vi "Host - Thruster Decode (SubVI).vi"(10 "Array":dbl[](array[numeric])=[0.0, 0.0, 0.0, 0.0, 0.0, 0.0, 0.0, 0.0, 0.0, 0.0, 0.0], 11 "read buffer":string) -> (3 "Data init out":dbl[](array[numeric]))   [LabVIEW 2021]
panel:
  out "thruster data":dbl[](array[numeric])
  out "speed":dbl
  out "command 55":u8[](array[numeric])
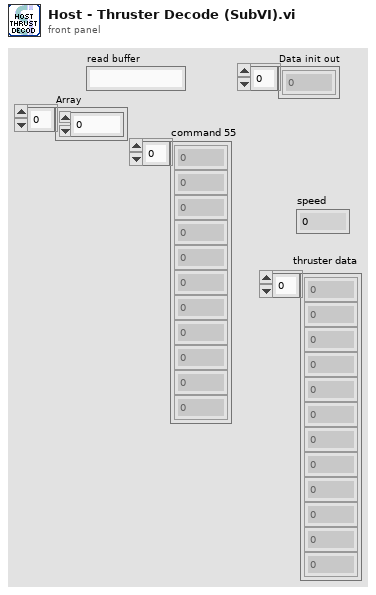
[diagram p1: front panel]
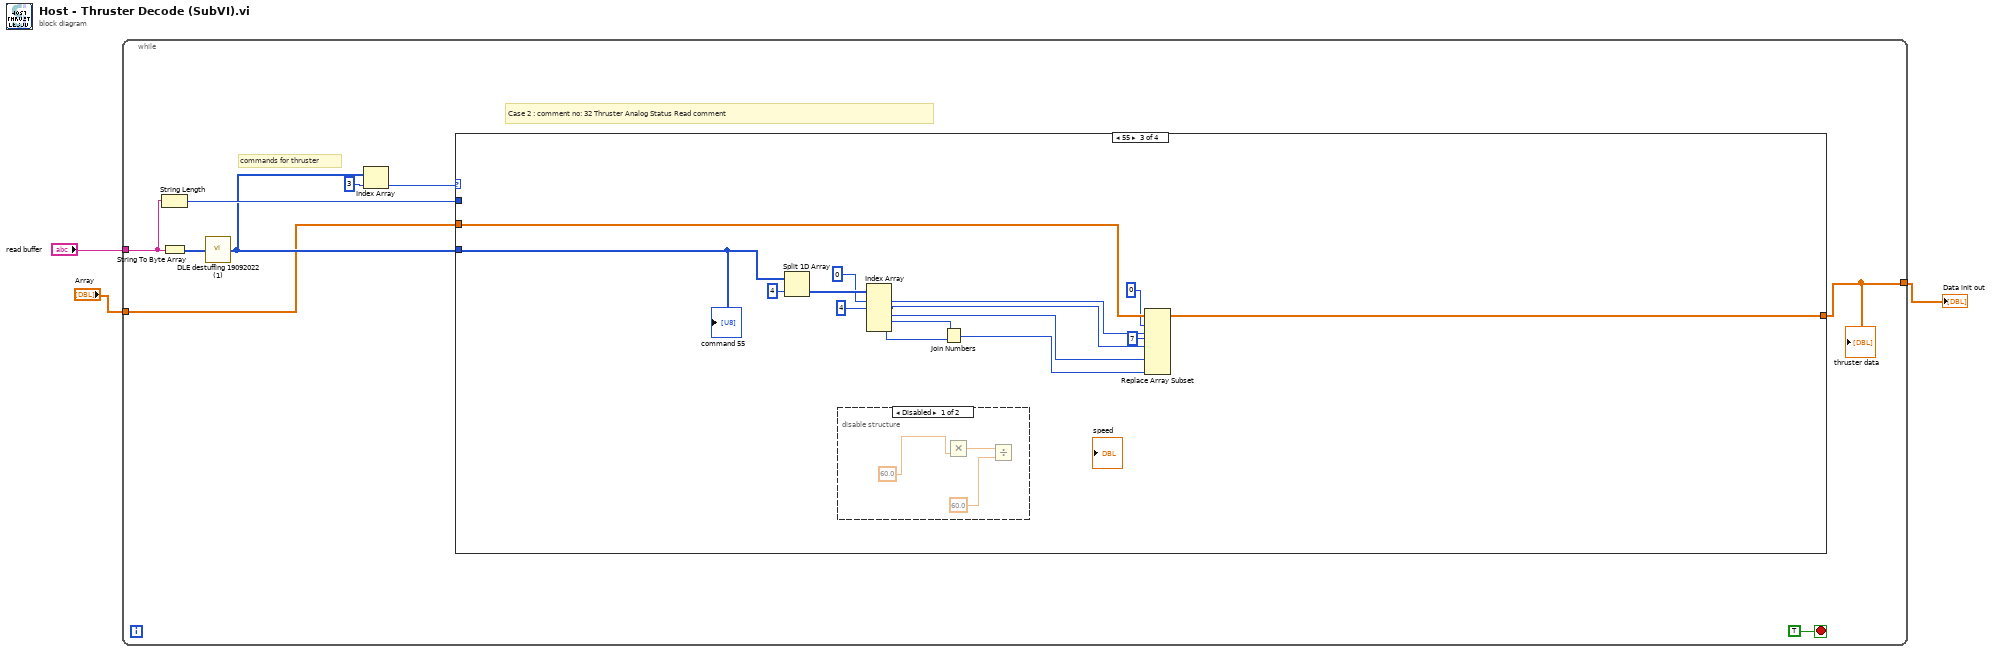
[diagram p0: block diagram]
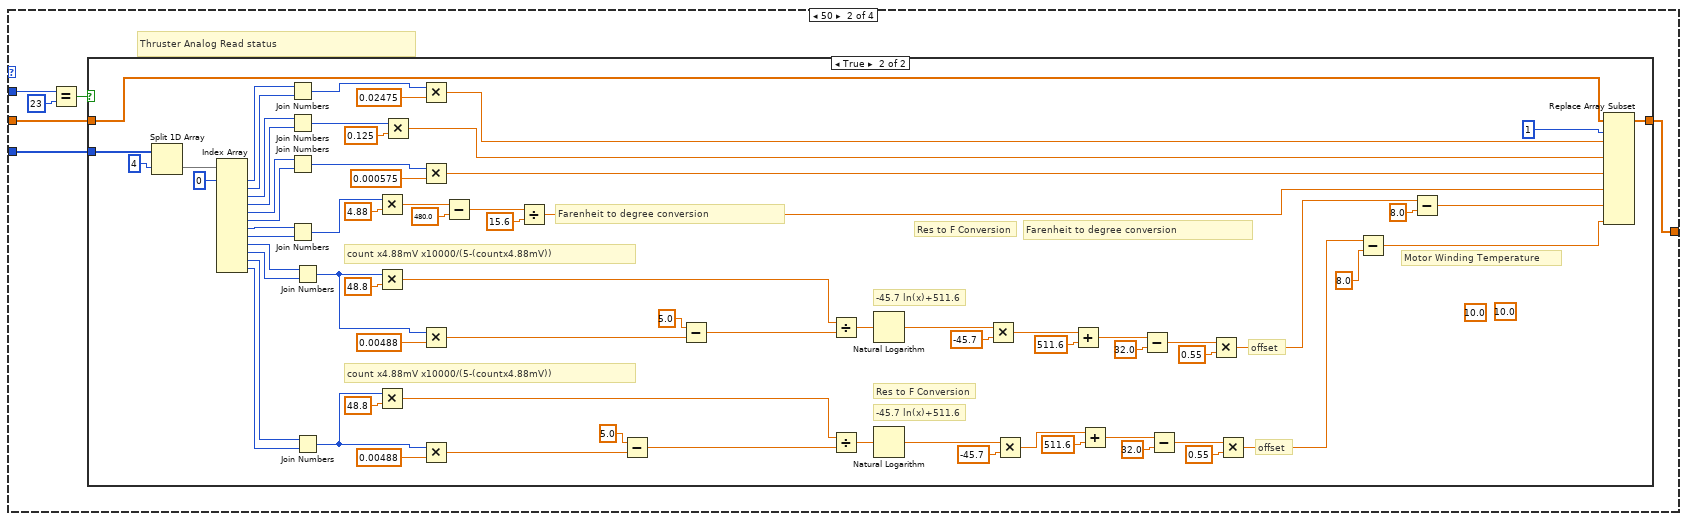
[diagram p3: hidden frame]
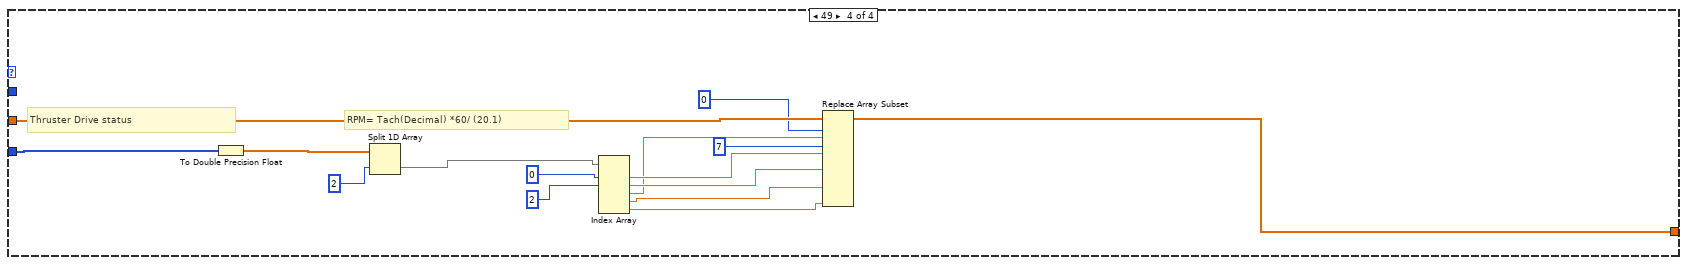
[diagram p6: hidden frame]
diagram:
  n1 = while {
    tunnel: "read buffer" -> [w4]
    tunnel: [w6] -> w2
    tunnel: "Array" -> [w5]
    stop <- TRUE stop-if-true
    # "commands for thruster"
    # "Case 2 : comment no: 32 Thruster Analog Status Read comment"
    n2 = String Length(string=w4) -> (length=w12:i32)
    n3 = String To Byte Array(string=w4) -> (unsigned byte array=w10:u8[])
    n4 = call "DLE destuffing 19092022 (1).vi"("DLE stuffed input"=w10) -> ("DLE destuffed output"=w11:u8[])  [unwired: 4 in]
    n5 = Index Array(array=w11, index=3) -> (element=w8:u8)
    n6 = case shown="55" w8 {
      tunnel: w11 -> [_ w19 w108 w113]
      tunnel: [w13 w17 w96 w125] -> w6
      tunnel: w5 -> [w13 w18 w101 w126]
      tunnel: w12 -> [_ w16 _ _]
      frame 0, Default {
      }
      frame 50 {
        # "Thruster Analog Read status"
        n7 = Equal?(x=w16, y=u32 23) -> (x = y?=w14:bool)
        n8 = case shown="True" w14 {
          tunnel: w19 -> [_ w93]
          tunnel: w18 -> [w20 w30]
          tunnel: [w20 w25] -> w17
          frame False {
          }
          frame True {
            (unwired) 10.0 ("y")
            (unwired) 10.0 ("y")
            # "offset"
            # "-45.7 ln(x)+511.6"
            # "Motor Winding Temperature"
            # "offset"
            # "-45.7 ln(x)+511.6"
            # "Farenheit to degree conversion"
            # "Res to F Conversion"
            # "count x4.88mV x10000/(5-(countx4.88mV))"
            # "Farenheit to degree conversion"
            # "Res to F Conversion"
            # "count x4.88mV x10000/(5-(countx4.88mV))"
            n9 = Split 1D Array(array=w93, index=4) -> (second subarray=w24:u8[])  [unwired: 1 out]
            n10 = Index Array(array=w24, index #1=0 ("index")) -> (element #1=w90:u8, element #2=w89:u8, element #3=w88:u8, element #4=w87:u8, element #5=w86:u8, element #6=w85:u8, element #7=w84:u8, element #8=w83:u8, element #9=w82:u8, element #10=w81:u8, element #11=w80:u8, element #12=w79:u8)  [unwired: 11 in]
            n11 = Join Numbers(hi=w90, lo=w89) -> ((hi.lo)=w78:u16)
            n12 = Join Numbers(hi=w88, lo=w87) -> ((hi.lo)=w76:u16)
            n13 = Join Numbers(hi=w86, lo=w85) -> ((hi.lo)=w74:u16)
            n14 = Join Numbers(hi=w84, lo=w83) -> ((hi.lo)=w72:u16)
            n15 = Join Numbers(hi=w82, lo=w81) -> ((hi.lo)=w32:u16)
            n16 = Join Numbers(hi=w80, lo=w79) -> ((hi.lo)=w31:u16)
            n17 = Multiply(x=w72, y=4.88) -> (x*y=w70:dbl)
            n18 = Multiply(x=w32, y=48.8) -> (x*y=w52:dbl)
            n19 = Multiply(x=w31, y=48.8) -> (x*y=w35:dbl)
            n20 = Multiply(x=w76, y=0.125) -> (x*y=w23:dbl)
            n21 = Multiply(x=w78, y=0.02475) -> (x*y=w22:dbl)
            n22 = Multiply(x=w74, y=0.000575) -> (x*y=w28:dbl)
            n23 = Multiply(x=w32, y=0.00488) -> (x*y=w63:dbl)
            n24 = Multiply(x=w31, y=0.00488) -> (x*y=w46:dbl)
            n25 = Subtract(x=w70, y=480.0) -> (x-y=w68:dbl)
            n26 = Divide(x=w68, y=15.6) -> (x/y=w21:dbl)
            n27 = Subtract(x=5.0, y=w46) -> (x-y=w47:dbl)
            n28 = Subtract(x=5.0, y=w63) -> (x-y=w64:dbl)
            n29 = Divide(x=w52, y=w64) -> (x/y=w58:dbl)
            n30 = Divide(x=w35, y=w47) -> (x/y=w41:dbl)
            n31 = Natural Logarithm(1:w58) -> (0:w57:dbl)
            n32 = Natural Logarithm(1:w41) -> (0:w40:dbl)
            n33 = Multiply(x=w57, y=-45.7) -> (x*y=w55:dbl)
            n34 = Multiply(x=w40, y=-45.7) -> (x*y=w38:dbl)
            n35 = Add(x=w55, y=511.6) -> (x+y=w53:dbl)
            n36 = Add(x=w38, y=511.6) -> (x+y=w36:dbl)
            n37 = Subtract(x=w53, y=32.0) -> (x-y=w60:dbl)
            n38 = Subtract(x=w36, y=32.0) -> (x-y=w43:dbl)
            n39 = Multiply(x=w60, y=0.55) -> (x*y=w51:dbl)
            n40 = Multiply(x=w43, y=0.55) -> (x*y=w34:dbl)
            n41 = Subtract(x=w34, y=8.0) -> (x-y=w26:dbl)
            n42 = Subtract(x=w51, y=8.0) -> (x-y=w27:dbl)
            n43 = Replace Array Subset(array=w30, new element #1=w22, index #1=1 ("index"), new element #2=w23, new element #3=w28, new element #4=w21, new element #5=w27, new element #6=w26) -> (w25:dbl[])  [unwired: 5 in]
          }
        }
      }
      frame 55 {
        n44 = Split 1D Array(array=w108, index=4) -> (second subarray=w106:u8[])  [unwired: 1 out]
        n45 = disable-structure shown="Disabled" {
          frame Disabled {
            n46 = Multiply(y=60.0) -> (x*y=w110:dbl)  [unwired: 1 in]
            n47 = Divide(x=w110, y=60.0) -> ()  [unwired: 1 out]
          }
          frame Enabled {
          }
        }
        n48 = Index Array(array=w106, index #1=0 ("index"), index #2=4 ("index")) -> (element #1=w99:u8, element #2=w98:u8, element #3=w97:u8, element #4=w103:u8, element #5=w102:u8)  [unwired: 3 in]
        n49 = Join Numbers(hi=w103, lo=w102) -> ((hi.lo)=w94:u16)
        n50 = Replace Array Subset(array=w101, new element #1=w99, index #1=0 ("index"), new element #2=w98, index #2=7 ("index"), new element #3=w97, new element #4=w94) -> (w96:dbl[])  [unwired: 2 in]
        "command 55" <- w108
      }
      frame 49 {
        # "RPM= Tach(Decimal) *60/ (20.1)"
        # "Thruster Drive status"
        n51 = To Double Precision Float(number=w113) -> (double precision float=w112:dbl[])
        n52 = Split 1D Array(array=w112, index=2) -> (second subarray=w124:dbl[])  [unwired: 1 out]
        n53 = Index Array(array=w124, index #1=0 ("index"), index #2=2 ("index")) -> (element #1=w120:dbl, element #2=w117:dbl, element #3=w114:dbl, element #4=w116:dbl, element #5=w115:dbl)  [unwired: 3 in]
        n54 = Replace Array Subset(array=w126, new element #1=w120, index #1=0 ("index"), new element #2=w117, index #2=7 ("index"), new element #3=w114, new element #4=w116, new element #5=w115) -> (w125:dbl[])  [unwired: 3 in]
      }
    }
    "thruster data" <- w6
  }
  "Data init out" <- w2
